vi "Get ni_measurementlink_measurement_v1_MeasureRequest.vi"(8 "error in (no error)":errorcluster, 11 "gRPCid":T1) -> (0 "error out":errorcluster, 2 "package_templatemessage":T2, 3 "gRPCid out":T1)   [LabVIEW 2020, in "Measurement Plugin Measurement Server Internal.lvlib"]
uses:
  Measurement Plugin Measurement Server Internal.lvlib
  ni_measurementlink_measurement_v1_MeasureRequest.ctl
  google_protobuf_Any.ctl
  ni_measurementlink_PinMapContext.ctl
  <vilib>/gRPC/LabVIEW gRPC Library/Shared/grpcId.ctl
  ni_measurementlink_measurement_v1_MeasureRequest_Flat.ctl
  google_protobuf_Any_Flat.ctl
  ni_measurementlink_PinMapContext_Flat.ctl
  2ed25e12-861d-4677-8ead-ace2906b2041.vi
  <vilib>/gRPC/LabVIEW gRPC Library/Shared/TranslateGrpcError.vi
  FlatToRichgoogle_protobuf_Any.vi
  FlatToRichni_measurementlink_PinMapContext.vi
  <vilib>/gRPC/LabVIEW gRPC Library/Server API/Server/Get Server DLL Path.vi
  <vilib>/Utility/error.llb/Error Cluster From Error Code.vi
  <vilib>/Utility/error.llb/Simple Error Handler.vi
  <vilib>/gRPC/LabVIEW gRPC Library/grpc-lvsupport-release.lvlib
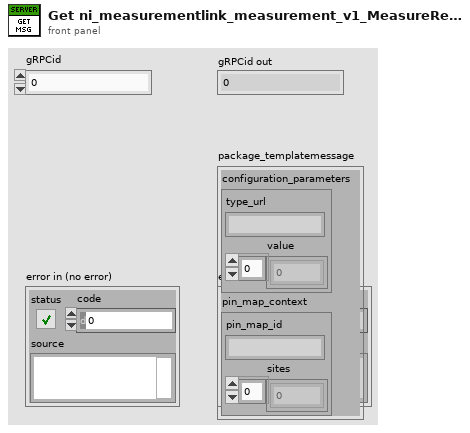
[diagram p1: front panel]
types:
  T1 = typedef "grpc-lvsupport-release.lvlib/grpcId.ctl" = u64
  T2 = typedef "Measurement Plugin Measurement Server Internal.lvlib/ni_measurementlink_measurement_v1_MeasureRequest.ctl" = cluster{"configuration_parameters":T3, "pin_map_context":T4}
  T3 = typedef "Measurement Plugin Measurement Server Internal.lvlib/google_protobuf_Any.ctl" = cluster{"type_url":string, "value":u8[]}
  T4 = typedef "Measurement Plugin Measurement Server Internal.lvlib/ni_measurementlink_PinMapContext.ctl" = cluster{"pin_map_id":string, "sites":i32[]}
  T5 = typedef "Measurement Plugin Measurement Server Internal.lvlib/ni_measurementlink_measurement_v1_MeasureRequest_Flat.ctl" = cluster{"configuration_parameters":T6, "pin_map_context":T7}
  T6 = typedef "Measurement Plugin Measurement Server Internal.lvlib/google_protobuf_Any_Flat.ctl" = cluster{"type_url":string, "value":u8[]}
  T7 = typedef "Measurement Plugin Measurement Server Internal.lvlib/ni_measurementlink_PinMapContext_Flat.ctl" = cluster{"pin_map_id":string, "sites":i32[]}
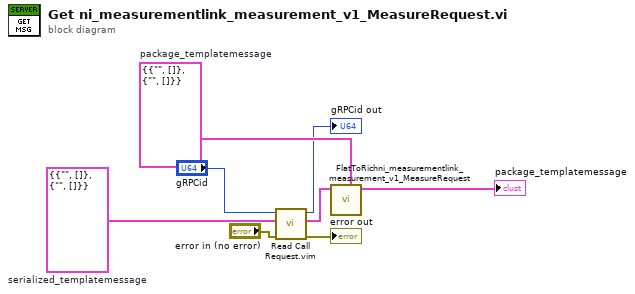
[diagram p0: block diagram]
diagram:
  w6 = T5 {"configuration_parameters"={"type_url"="", "value"=[]}, "pin_map_context"={"pin_map_id"="", "sites"=[]}}  # serialized_templatemessage
  w5 = T2 {"configuration_parameters"={"type_url"="", "value"=[]}, "pin_map_context"={"pin_map_id"="", "sites"=[]}}  # package_templatemessage
  n1 = call "Read Call Request.vim"("error in"="error in (no error)", "Request Type"=w6, "gRPCid in"="gRPCid") -> ("error out"=→"error out":errorcluster, "Request Data"=w4:T5, "gRPCid out"=→"gRPCid out":T1)  [unwired: 6 in]
  n2 = call "FlatToRichni_measurementlink_measurement_v1_MeasureRequest.vi"("OutputClusterType"=w5, "InputCluster"=w4) -> ("OutputCluster"=→"package_templatemessage":T2)  [unwired: 9 in]
